vi "Agilent E4980 Read Measurement.vi"() -> ()   [LabVIEW 2017]
doc: "This example shows how to configure a measurement and take readings."
uses:
  <vilib>/Platform/TimedLoop/XDataNode/timing_clust.ctl
  <vilib>/Platform/TimedLoop/XDataNode/nitl_modes.ctl
  <vilib>/Platform/TimedLoop/XDataNode/wakeup.ctl
  <vilib>/platform/TimedLoop/XDataNode/XDataNode.xnode
  Agilent E4980.lvlib
  <vilib>/Platform/TimedLoop/XDataNode/XDNodeRunTimeDep.lvlib
panel:
  in  "Stop Button":bool
  in  "file path (use dialog)":path
  out "Secondary":dbl(graph)
  out "Primary":dbl(graph)
  in  "Averaging Factor (1)":i32=1
  in  "Measurement Time (1: Medium)":u16(ring)=1 items=["Short", "Medium", "Long"]
  in  "Signal Level (1.0 V)":dbl=1.0
  in  "Signal Type (0: Voltage)":u16(ring) items=["Voltage", "Current"]
  in  "Signal Frequency (1000 Hz)":dbl=1000.0
  in  "Enable Auto Range (T:Enable)":bool=TRUE
  in  "Manual Impedance Range (3: 100 Ohms)":i32(ring)=3 items=["100m", "1", "10", "100", "300", "1K", "3K", "10K", "30K", "100K"]
  in  "Function (0: Cp-D)":u16(ring) items=["Cp-D", "Cp-Q", "Cp-G", "Cp-Rp", "Cs-D", "Cs-Q", "Cs-Rs", "Lp-D", "Lp-Q", "Lp-G", "Lp-Rp", "Lp-Rdc", "Ls-D", "Ls-Q", "Ls-Rs", "Ls-Rdc", "R-X", "Z-thd", "Z-thr", "G-B", "Y-thd", "Y-thr", "Vdc-Idc"]
  in  "VISA resource name":refnum<visa-resource-name>
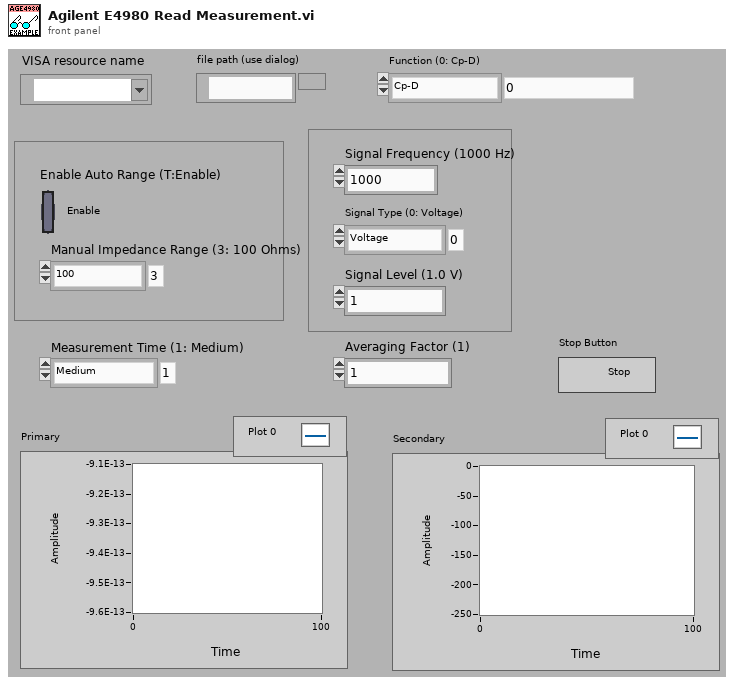
[diagram p1: front panel]
types:
  T1 = typedef "XDNodeRunTimeDep.lvlib/timing_clust.ctl" = cluster{"Expected End [f-1]":u64, "Actual End [f-1]":u64, "Finished Late? [f-1]":bool, "Expected End [i-1]":u64, "Actual End [i-1]":u64, "Finished Late? [i-1]":bool, "Expected Start [i]":u64, "Actual Start [i]":u64, "Expected Start [f]":u64, "Actual Start [f]":u64, "Source Name":string, "Structure Name":string, "Period":i64, "Deadline":i64, "Offset":i64, "Start":i64, "Priority":i32, "Timeout":i32, "Mode":T2, "Wakeup Reason":T3, "Error":errorcluster, "Source Type":string, "Secondary Source Type":string, "Global End Time":u64, "Global Start Time":u64, "Frame Duration":u64, "Iteration Duration":u64, "Assigned CPU":i32, "I/O Scan Engine Mode":u32}
  T2 = typedef "XDNodeRunTimeDep.lvlib/nitl_modes.ctl" = enum32{"No Change", "Process missed periods, maintain original phase", "Discard missed periods, maintain original phase", "Process missed periods, ignore original phase", "Discard missed periods, ignore original phase"}
  T3 = typedef "XDNodeRunTimeDep.lvlib/wakeup.ctl" = enum32{"Normal", "Aborted", "Asynchronous wakeup", "Timing source error", "Timed loop error", "Timeout"}
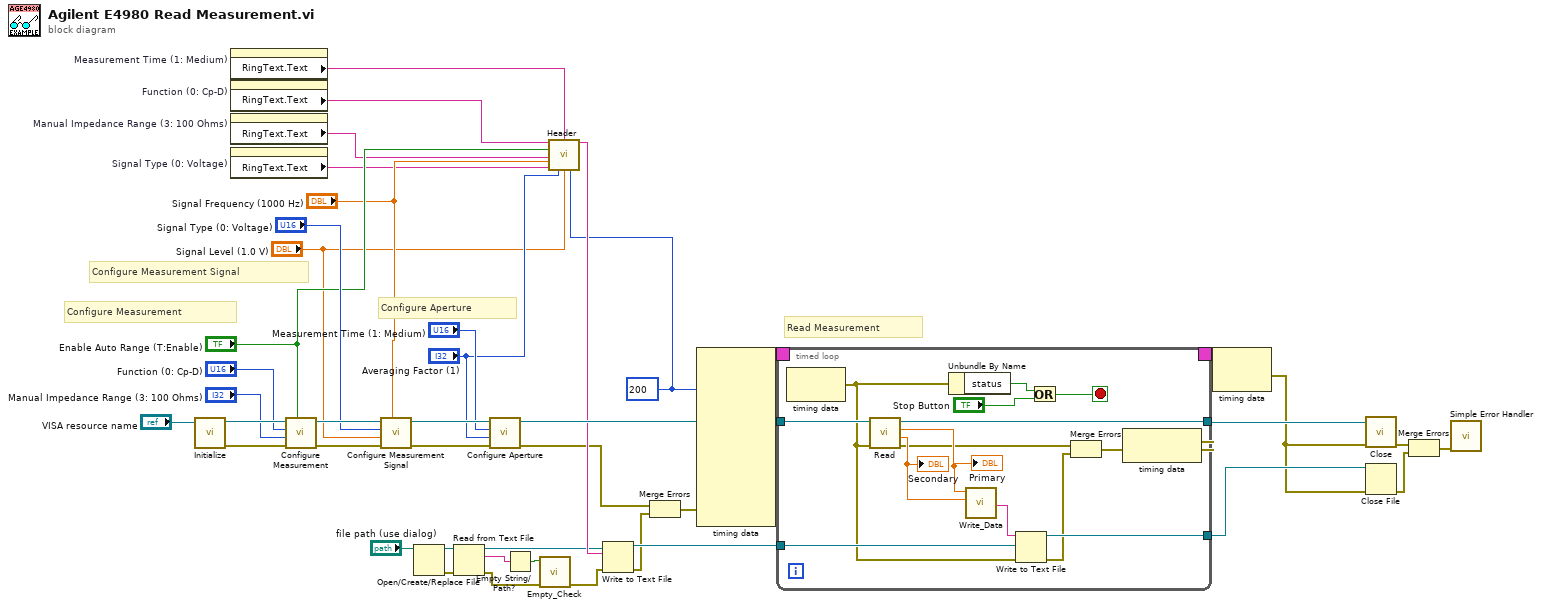
[diagram p0: block diagram]
diagram:
  w1 = 200
  # "Configure Aperture"
  # "Configure Measurement Signal"
  # "Read Measurement"
  # "Configure Measurement"
  n1 = call "Initialize.vi"("VISA resource name"="VISA resource name") -> ("error out"=w40:errorcluster, "VISA resource name out"=w41:refnum<visa-resource-name>)  [unwired: 9 in]
  n2 = property on="Measurement Time (1: Medium)" class="Ring (strict)"() -> ("RingText.Text"=w7:string)  [unwired: 2 in, 2 out]
  n3 = property on="Function (0: Cp-D)" class="Ring (strict)"() -> ("RingText.Text"=w25:string)  [unwired: 2 in, 2 out]
  n4 = property on="Manual Impedance Range (3: 100 Ohms)" class="Ring (strict)"() -> ("RingText.Text"=w23:string)  [unwired: 2 in, 2 out]
  n5 = property on="Signal Type (0: Voltage)" class="Ring (strict)"() -> ("RingText.Text"=w21:string)  [unwired: 2 in, 2 out]
  n6 = call "Configure Measurement.vi"("Enable Auto Range (T:Enable)"="Enable Auto Range (T:Enable)", "error in (no error)"=w40, "Manual Impedance Range (3: 100 Ohms)"="Manual Impedance Range (3: 100 Ohms)", "Function (0: Cp-D)"="Function (0: Cp-D)", "VISA resource name"=w41) -> ("error out"=w38:errorcluster, "VISA resource name out"=w39:refnum<visa-resource-name>)  [unwired: 5 in]
  n7 = call "Configure Measurement Signal.vi"("Signal Frequency (1000 Hz)"="Signal Frequency (1000 Hz)", "error in (no error)"=w38, "Signal Level (1.0 V)"="Signal Level (1.0 V)", "Signal Type (0: Voltage)"="Signal Type (0: Voltage)", "VISA resource name"=w39) -> ("error out"=w36:errorcluster, "VISA resource name out"=w37:refnum<visa-resource-name>)  [unwired: 5 in]
  n8 = Open/Create/Replace File(file path (use dialog)="file path (use dialog)") -> (refnum out=w16:refnum<file>, error out=w13:errorcluster)  [unwired: 5 in, 1 out]
  n9 = Read from Text File(file (use dialog)=w16, error in=w13) -> (refnum out=w14:refnum<file>, text=w17:string, error out=w12:errorcluster)  [unwired: 2 in, 1 out]
  n10 = call "Configure Aperture.vi"("error in (no error)"=w36, "Averaging Factor (1)"="Averaging Factor (1)", "Measurement Time (1: Medium)"="Measurement Time (1: Medium)", "VISA resource name"=w37) -> ("error out"=w10:errorcluster, "VISA resource name out"=w29:refnum<visa-resource-name>)  [unwired: 6 in]
  n11 = Empty String/Path?(string/path=w17) -> (empty?=w15:bool)
  n12 = call "Empty_Check.vi"("error in (no error)"=w12, "Boolean"=w15) -> ("error out"=w11:errorcluster)  [unwired: 9 in]
  n13 = call "Header.vi"("Function"=w25, "Measurement Time"=w7, "Auto Range"="Enable Auto Range (T:Enable)", "Manual Impedance Range"=w23, "Signal Frequency"="Signal Frequency (1000 Hz)", "Signal Type"=w21, "Averaging Factor"="Averaging Factor (1)", "Signal Level"="Signal Level (1.0 V)", "dt"=w1) -> ("Header"=w18:string)  [unwired: 6 in]
  n14 = Write to Text File(file (use dialog)=w14, text=w18, error in=w11) -> (refnum out=w19:refnum<file>, error out=w9:errorcluster)  [unwired: 1 in, 1 out]
  n15 = Merge Errors(w10, w9) -> (w8:errorcluster)
  n16 = node-c288(w1, w8) -> (w31:T1)  [unwired: 8 in]
  n17 = timed-loop {
    timing: w31 -> [_]
    timing-out: [_] -> w30
    tunnel: w29 -> [w56]
    tunnel: [w55] -> w28
    tunnel: w19 -> [w52]
    tunnel: [w53] -> w26
    stop <- w49 stop-if-true
    n18 = node-c288() -> (w46:errorcluster)  [unwired: 1 in]
    n19 = call "Read.vi"("error in (no error)"=w46, "VISA resource name"=w56) -> ("error out"=w45:errorcluster, "Secondary Parameter"=w54:dbl, "Primary Parameter"=w50:dbl, "VISA resource name out"=w55:refnum<visa-resource-name>)  [unwired: 6 in]
    "Primary" <- w50
    "Secondary" <- w54
    n20 = Unbundle By Name(w46) -> ("status"=w48:bool)
    n21 = call "Write_Data.vi"("Secondary Parameter"=w54, "Primary Parameter"=w50) -> ("String"=w51:string)  [unwired: 9 in]
    n22 = Write to Text File(file (use dialog)=w52, text=w51, error in=w46) -> (refnum out=w53:refnum<file>, error out=w44:errorcluster)  [unwired: 1 in, 1 out]
    n23 = Or(x=w48, y="Stop Button") -> (x .or. y?=w49:bool)
    n24 = Merge Errors(w45, w44) -> (w43:errorcluster)
    n25 = node-c288(w43) -> ()  [unwired: 1 out]
  }
  n26 = node-c288(w30) -> (w6:errorcluster)
  n27 = call "Close.vi"("error in (no error)"=w6, "VISA resource name"=w28) -> ("error out"=w4:errorcluster)  [unwired: 9 in]
  n28 = Close File(refnum=w26, error in=w6) -> (error out=w5:errorcluster)  [unwired: 1 out]
  n29 = Merge Errors(w4, w5) -> (w3:errorcluster)
  n30 = call <vilib>:"Simple Error Handler.vi"("error in (no error)"=w3) -> ()  [unwired: 4 in, 5 out]
